vi "Value of Time.vi"(2 "input file":refnum<file>, 3 "error in":errorcluster) -> (0 "output file refnum":refnum<file>, 1 "error out":errorcluster)   [LabVIEW 2018]
doc: "Производится запись временеи (даты) и запись мирового компьютерного времени в текстовый файл"
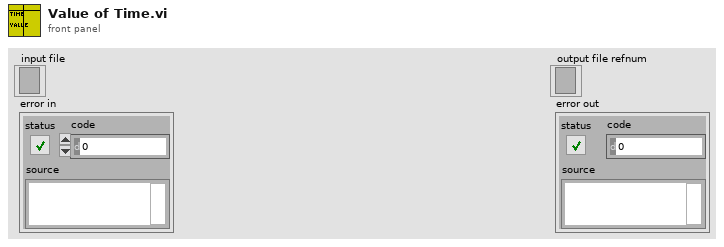
[diagram p1: front panel]
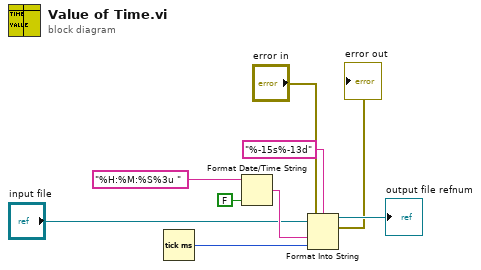
[diagram p0: block diagram]
diagram:
  n1 = Tick Count (ms)() -> (millisecond timer value=w6:u32)
  n2 = Format Date/Time String(time format string (%c)="%H:%M:%S%3u ", UTC format=FALSE) -> (date/time string=w7:string)  [unwired: 1 in]
  n3 = Format Into String(format string="%-15s%-13d", initial string="input file", error in="error in", w7, w6) -> (resulting string=→"output file refnum":refnum<file>, error out=→"error out":errorcluster)
